vi "Close M3102A.vi"(8 "errorIn":errorcluster, 11 "moduleID":i32) -> (0 "errorOut":errorcluster)   [LabVIEW 2020]
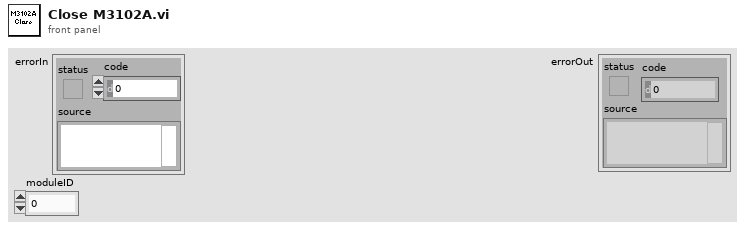
[diagram p1: front panel]
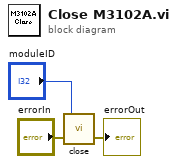
[diagram p0: block diagram]
diagram:
  n1 = call <vilib>:"close.vi"("errorIn"="errorIn", "moduleID"="moduleID") -> ("errorOut"=→"errorOut":errorcluster)  [unwired: 1 in]
